vi "Global Teardown.vi"(8 "error in (no error)":errorcluster, 11 "Global Fixture Test Case in":refnum<class "Global Fixture Test Case.lvclass">) -> (0 "error out":errorcluster)   [LabVIEW 2020, in "Global Fixture Test Case.lvclass"]
uses:
  Global Fixture Test Case.lvclass
  Global Fixture Test Case.lvclass/Global Fixture Test Case.ctl
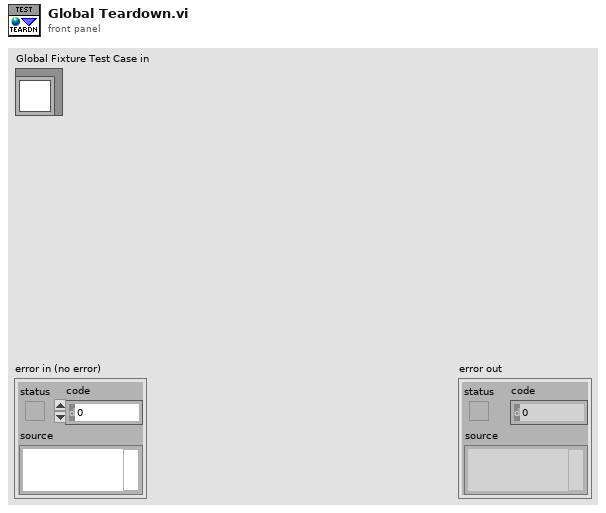
[diagram p1: front panel]
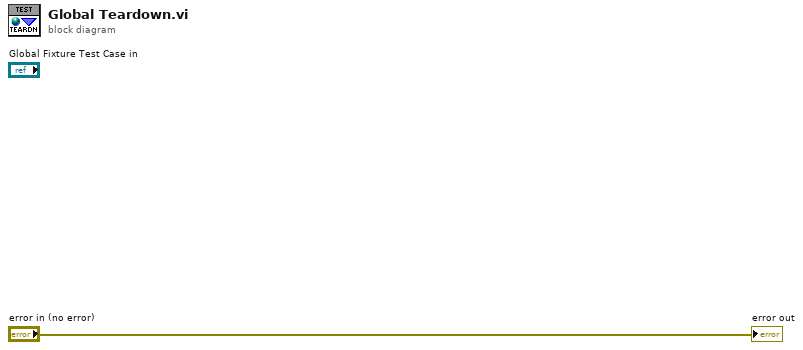
[diagram p0: block diagram]
diagram:
  "error out" <- "error in (no error)"
